vi "Add Item to Tree.vi"(8 "error in (no error)":errorcluster, 10 "Express VI Type in":refnum<class "Express VI Type.lvclass">, 11 "Tree Ref in":refnum<vi>) -> (0 "error out":errorcluster, 1 "Added Tag":string, 2 "Express VI Type out":refnum<class "Express VI Type.lvclass">, 3 "Tree Ref out":refnum<vi>)   [LabVIEW 2020, in "Peek Window.lvlib" / "Express VI Type.lvclass"]
uses:
  Express VI Type.lvclass
  Symbols Enum.ctl
  Express VI Type.lvclass/Express VI Type.ctl
  Standard VI Type/Standard VI Type.lvclass/Standard VI Type.ctl
  Standard VI Type/Read Full Qualified Name.vi
  Implementation VI Type/Implementation VI Type.lvclass
  D:/Code/VI-Peek/source/Peek Window/VI Types/Standard VI Type/Standard VI Type.lvclass
  Peek Window.lvlib
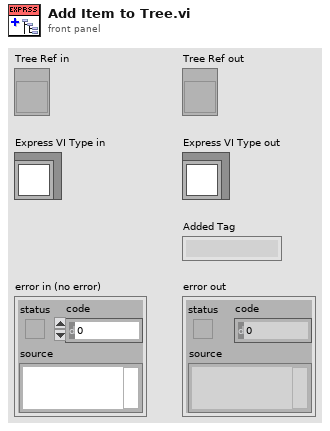
[diagram p1: front panel]
types:
  T1 = typedef "Peek Window.lvlib/Symbols Enum.ctl" = enum16{"<Blank>", "Below Here Glyph", "VI", "Dynamic Dispatch VI", "Malleable VI", "Polymorphic VI", "Missing VI", "Express VI"}
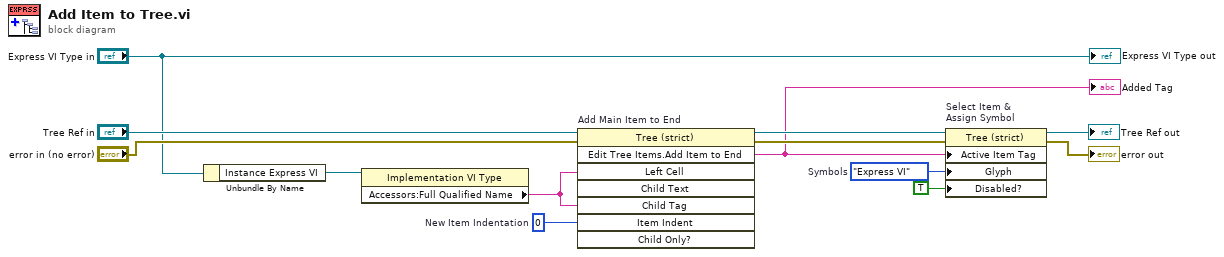
[diagram p0: block diagram]
diagram:
  w7 = Symbols_Enum."Express VI"  # Symbols
  w13 = 0  # New Item Indentation
  n1 = Unbundle By Name("Express VI Type in") -> ("Instance Express VI"=w6:refnum<class "Implementation VI Type.lvclass">)
  n2 = property class="Implementation VI Type"(reference=w6) -> ("Accessors:Full Qualified Name"=w2:string)  [unwired: 1 in, 2 out]
  n3 = invoke on="Add Main Item to End" class="Tree (strict)" method="Edit Tree Items.Add Item to End"(reference="Tree Ref in", error in="error in (no error)", "Left Cell"=w2, "Child Tag"=w2, "Item Indent"=w13) -> (reference out=w10:refnum<vi>, error out=w9:errorcluster, "Edit Tree Items:Add Item to End"=w8:string)  [unwired: 3 in, 5 out]
  "Added Tag" <- w8
  n4 = property on="Select Item &\nAssign Symbol" class="Tree (strict)"(reference=w10, error in=w9, "Active Item Tag"=w8, "Glyph"=w7, "Disabled?"=TRUE) -> (reference out=→"Tree Ref out":refnum<vi>, error out=→"error out":errorcluster)
  "Express VI Type out" <- "Express VI Type in"
